vi "Build.vi"(6 "ItemBuilt":T1, 8 "error in (no error)":errorcluster, 11 "BuildManager in":refnum<class "BuildManager.lvclass">) -> (0 "error out":errorcluster, 3 "BuildManager out":refnum<class "BuildManager.lvclass">)   [LabVIEW 2020, in "SolutionBuilder.lvlib" / "BuildManager.lvclass"]
uses:
  BuildManager.lvclass
  Events/EventItemBuilt.ctl
  BuildManager.lvclass/BuildManager.ctl
  ProjectItem/ProjectItem.lvclass
  SolutionBuilder.lvlib
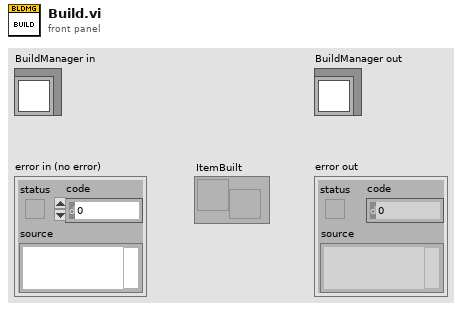
[diagram p1: front panel]
types:
  T1 = typedef "SolutionBuilder.lvlib/EventItemBuilt.ctl" = refnum<user-event>
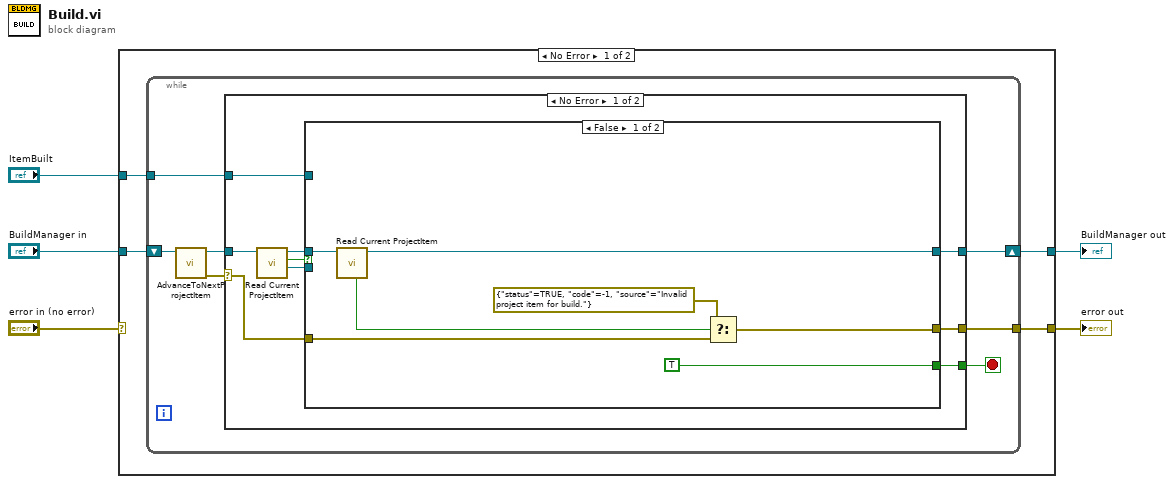
[diagram p0: block diagram]
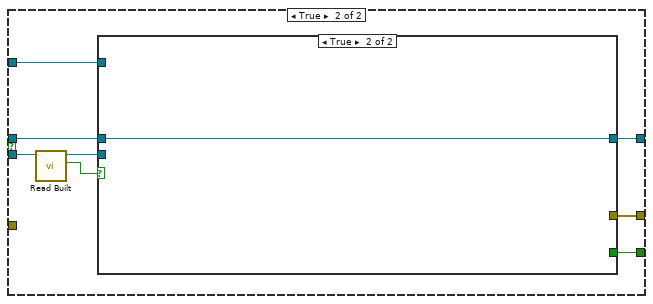
[diagram p2: hidden frame]
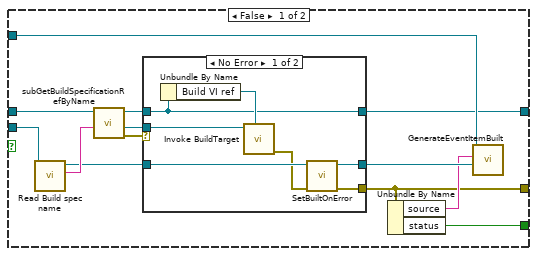
[diagram p3: hidden frame]
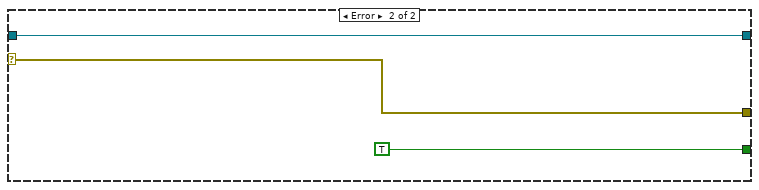
[diagram p5: hidden frame]
diagram:
  n1 = case shown="No Error" "error in (no error)" {
    selector: "error in (no error)" -> [_ w69]
    tunnel: "BuildManager in" -> [w9 w68]
    tunnel: "ItemBuilt" -> [w8 _]
    tunnel: [w6 w69] -> w2
    tunnel: [w7 w68] -> w1
    frame No Error {
      n2 = while {
        shift-right: [w14] -> w7
        shift-left: w9 -> [w16]
        tunnel: w8 -> [w12]
        tunnel: [w11] -> w6
        stop <- w13 stop-if-true
        n3 = call "AdvanceToNextProjectItem.vi"("BuildManager in"=w16) -> ("error out"=w10:errorcluster, "BuildManager out"=w15:refnum<class "BuildManager.lvclass">)  [unwired: 9 in]
        n4 = case shown="No Error" w10 {
          selector: w10 -> [w17 w65]
          tunnel: w15 -> [w25 w67]
          tunnel: [w21 w67] -> w14
          tunnel: [w20 TRUE ("status")] -> w13
          tunnel: w12 -> [w19 _]
          tunnel: [w18 w65] -> w11
          frame No Error {
            n5 = call-dynamic "Read Current ProjectItem.vi"("BuildManager in"=w25) -> ("Current ProjectItem"=w22:refnum<class "ProjectItem.lvclass">, "Valid"=w24:bool, "BuildManager out"=w23:refnum<class "BuildManager.lvclass">)  [unwired: 7 in, 1 out]
            n6 = case shown="False" w24 {
              tunnel: w23 -> [w30 w40]
              tunnel: w22 -> [_ w38]
              tunnel: [w31 w39] -> w21
              tunnel: [TRUE w34] -> w20
              tunnel: w19 -> [_ w35]
              tunnel: [w26 w33] -> w18
              tunnel: w17 -> [w27 _]
              frame False {
                n7 = call-dynamic "Read Current ProjectItem.vi"("BuildManager in"=w30) -> ("BuildManager out"=w31:refnum<class "BuildManager.lvclass">, "In bounds"=w29:bool)  [unwired: 7 in, 2 out]
                n8 = Select(t=errorcluster {"status"=TRUE, "code"=-1, "source"="Invalid project item for build."}, s=w29, f=w27) -> (s? t:f=w26:errorcluster)
              }
              frame True {
                n9 = call-dynamic "Read Built.vi"("ProjectItem in"=w38) -> ("Built"=w36:bool, "ProjectItem out"=w37:refnum<class "ProjectItem.lvclass">)  [unwired: 9 in]
                n10 = case shown="True" w36 {
                  tunnel: w40 -> [w53 w64]
                  tunnel: [w43 w64] -> w39
                  tunnel: w37 -> [w50 _]
                  tunnel: w35 -> [w47 _]
                  tunnel: [w45 _] -> w34
                  tunnel: [w41 _] -> w33
                  frame False {
                    n11 = call-dynamic "Read Build spec name.vi"("ProjectItem in"=w50) -> ("Build spec name"=w52:string, "ProjectItem out"=w49:refnum<class "ProjectItem.lvclass">)  [unwired: 9 in]
                    n12 = call "subGetBuildSpecificationRefByName.vi"("Name"=w52, "BuildManager in"=w53) -> ("error out"=w42:errorcluster, "Build spec ref"=w51:refnum<vi>, "BuildManager out"=w44:refnum<class "BuildManager.lvclass">)  [unwired: 7 in]
                    n13 = case shown="No Error" w42 {
                      selector: w42 -> [_ w61]
                      tunnel: w51 -> [w59 _]
                      tunnel: w49 -> [w58 w62]
                      tunnel: [w57 w62] -> w48
                      tunnel: [w55 w61] -> w41
                      tunnel: w44 -> [w54 w63]
                      tunnel: [w54 w63] -> w43
                      frame No Error {
                        n14 = Unbundle By Name(w54) -> ("Build VI ref"=w60:refnum<vi>)
                        n15 = call <vilib>:"Invoke BuildTarget.vi"("vi reference"=w60, "BuildItem ref"=w59) -> ("error out"=w56:errorcluster)  [unwired: 8 in, 1 out]
                        n16 = call "SetBuiltOnError.vi"("error in (no error)"=w56, "ProjectItem in"=w58) -> ("error out"=w55:errorcluster, "ProjectItem out"=w57:refnum<class "ProjectItem.lvclass">)  [unwired: 8 in]
                      }
                      frame Error {
                      }
                    }
                    n17 = Unbundle By Name(w41) -> ("source"=w46:string, "status"=w45:bool)
                    n18 = call "GenerateEventItemBuilt.vi"("ProjectItem"=w48, "Result"=w46, "ItemBuilt"=w47) -> ()  [unwired: 9 in]
                  }
                  frame True {
                  }
                }
              }
            }
          }
          frame Error {
          }
        }
      }
    }
    frame Error {
    }
  }
  "error out" <- w2
  "BuildManager out" <- w1
